vi "题目1.vi"   [LabVIEW 2017]
types:
  T1 = enum16{"open", "replace", "create", "open or create", "replace or create", "replace or create with confirmation"}
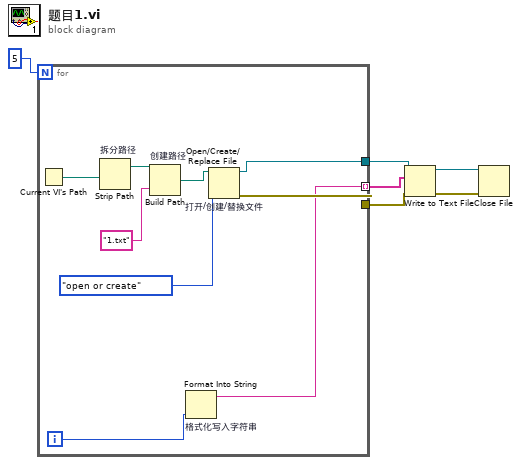
[diagram p0: block diagram]
diagram:
  n1 = for {
    N: 5 -> [_]
    tunnel: [w11] -> w3
    tunnel: [w10] -> w5
    tunnel: [w7] -> w4 mode=indexing
    i -> [w8]
    n2 = Current VI's Path() -> (path=w13:path)
    n3 = Strip Path "拆分路径"(path=w13) -> (stripped path=w15:path)  [unwired: 1 out]
    n4 = Build Path "创建路径"(base path=w15, name or relative path="1.txt" ("名称或相对路径")) -> (appended path=w14:path)
    n5 = Format Into String "格式化写入字符串"(w8) -> (resulting string=w7:string)  [unwired: 3 in, 1 out]
    n6 = Open/Create/Replace File "打开/创建/替换文件"(file path (use dialog)=w14, operation (0:open)=T1."open or create" ("操作(0:open)")) -> (refnum out=w10:refnum<file>, error out=w11:errorcluster)  [unwired: 4 in, 1 out]
  }
  n7 = Write to Text File(file (use dialog)=w5, text=w4, error in=w3) -> (refnum out=w2:refnum<file>, error out=w1:errorcluster)  [unwired: 1 in, 1 out]
  n8 = Close File(refnum=w2, error in=w1) -> ()  [unwired: 2 out]
